vi "TestExec.Print Label.vi"(5 "CfgItem":string="URLLabel1", 6 "URL":string, 7 "CfgSection":string="Printer", 8 "error in":errorcluster, 10 "Text to Print":string, 11 "Config File":path) -> (0 "error out":errorcluster)   [LabVIEW 2018]
uses:
  <vilib>/Utility/config.llb/Read Key (String).vi
  <vilib>/httpClient/LabVIEWHTTPClient.lvlib
  <vilib>/Utility/config.llb/NI_LVConfig.lvlib
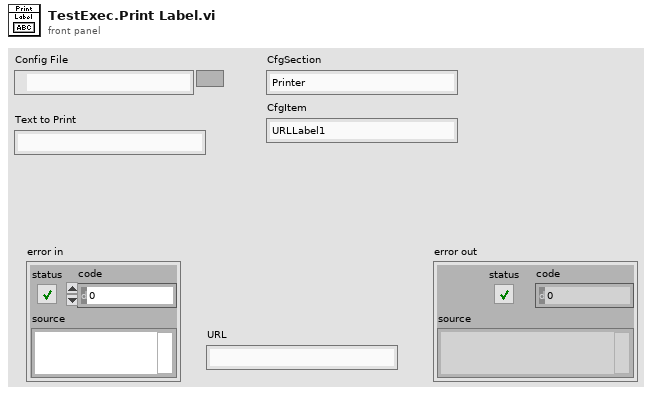
[diagram p1: front panel]
types:
  T1 = typedef "LabVIEWHTTPClient.lvlib/ClientHandle.ctl" = refnum<k1>
  T2 = typedef "NI_LVConfig.lvlib/Config Data RefNum.ctl" = refnum<k1>
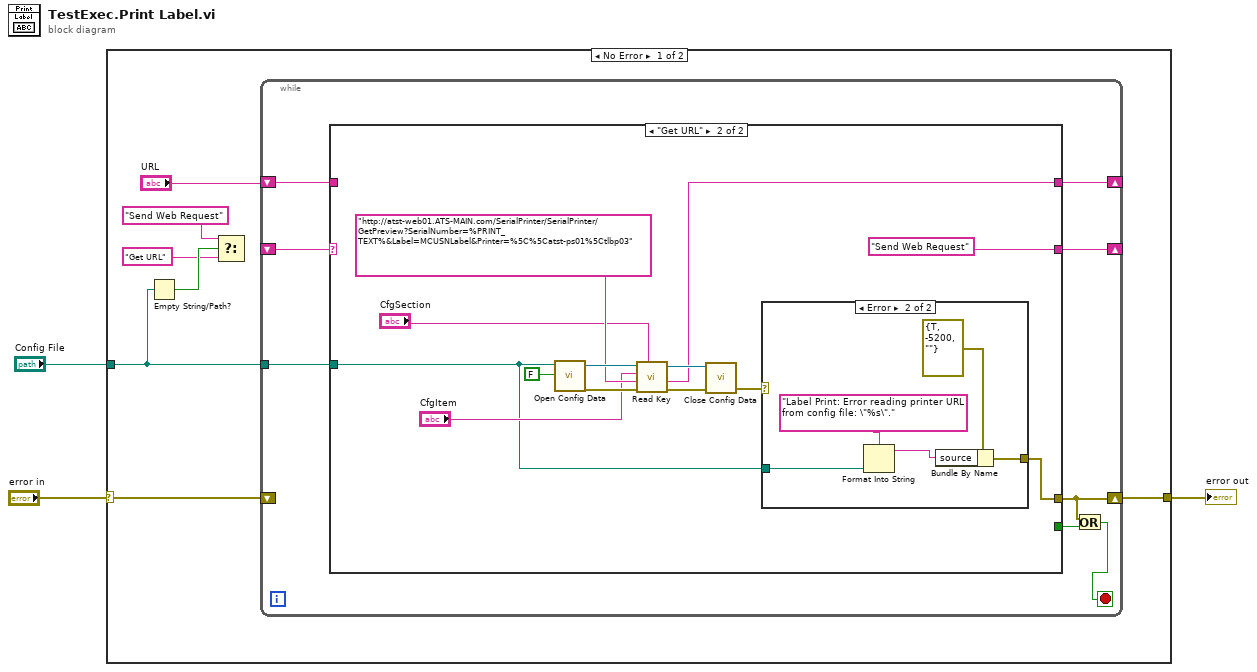
[diagram p0: block diagram]
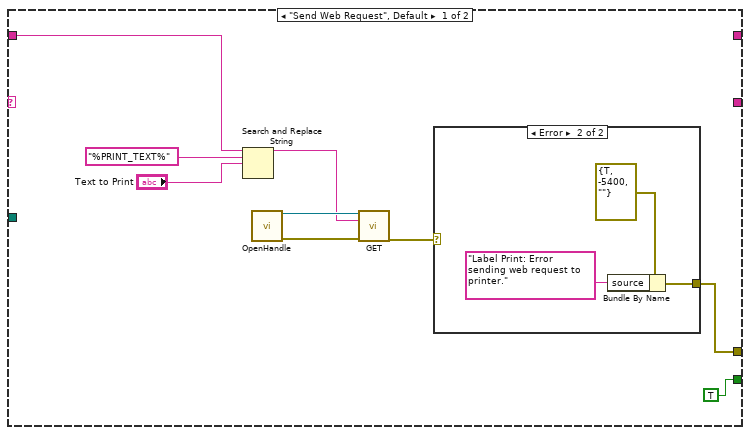
[diagram p2: hidden frame]
diagram:
  n1 = case shown="No Error" "error in" {
    selector: "error in" -> [w9 w49]
    tunnel: [w10 w49] -> w3
    tunnel: "Config File" -> [w6 _]
    frame No Error {
      n2 = Empty String/Path?(string/path=w6) -> (empty?=w7:bool)
      n3 = Select(t="Send Web Request", s=w7, f="Get URL") -> ()  [unwired: 1 out]
      n4 = while {
        shift-right: [w16] -> _
        shift-left: _ -> [w17]
        shift-right: [w15] -> _
        shift-left: "URL" -> [w18]
        shift-right: [w14] -> w10
        shift-left: w9 -> [_]
        tunnel: w6 -> [w11]
        stop <- w12 stop-if-true
        n5 = case shown="\"Get URL\"" w17 {
          tunnel: w18 -> [w26 _]
          tunnel: [_ "Send Web Request"] -> w16
          tunnel: [w20 w36] -> w14
          tunnel: [_ w35] -> w15
          tunnel: [TRUE _] -> w13
          tunnel: w11 -> [_ w31]
          frame "Send Web Request", Default {
            n6 = Search and Replace String(input string=w26, search string="%PRINT_TEXT%", replace string="Text to Print") -> (result string=w23:string)  [unwired: 5 in, 3 out]
            n7 = call <vilib>:"OpenHandle.vi"() -> ("client handle out"=w24:T1, "error out"=w25:errorcluster)  [unwired: 14 in]
            n8 = call <vilib>:"GET.vi"("client handle"=w24, "url"=w23, "error in (no error)"=w25) -> ("error out"=w21:errorcluster)  [unwired: 9 in, 3 out]
            n9 = case shown="Error" w21 {
              tunnel: [_ w29] -> w20
              frame No Error {
              }
              frame Error {
                n10 = Bundle By Name(cluster=errorcluster {"status"=TRUE, "code"=-5400, "source"=""} ("error constant"), "source"="Label Print: Error sending web request to printer.") -> (w29:errorcluster)
              }
            }
          }
          frame "Get URL" {
            n11 = call <vilib>:"Open Config Data.vi"("create file if necessary (T)"=FALSE, "configuration file path"=w31) -> ("error out"=w40:errorcluster, "refnum"=w41:T2)  [unwired: 7 in, 1 out]
            n12 = call-poly <vilib>:"Read Key.vi"("section"="CfgSection", "error in (no error)"=w40, "default value"="http://atst-web01.ATS-MAIN.com/SerialPrinter/SerialPrinter/GetPreview?SerialNumber=%PRINT_TEXT%&Label=MCUSNLabel&Printer=%5C%5Catst-ps01%5Ctlbp03", "key"="CfgItem", "refnum"=w41) -> ("error out"=w43:errorcluster, "value"=w35:string, "refnum out"=w42:T2)  [unwired: 3 in, 1 out]
            n13 = call <vilib>:"Close Config Data.vi"("error in (no error)"=w43, "refnum"=w42) -> ("error out"=w37:errorcluster)  [unwired: 8 in, 1 out]
            n14 = case shown="Error" w37 {
              tunnel: w31 -> [_ w45]
              tunnel: [_ w44] -> w36
              frame No Error {
              }
              frame Error {
                n15 = Format Into String(format string="Label Print: Error reading printer URL from config file: \"%s\".", w45) -> (resulting string=w46:string)  [unwired: 2 in, 1 out]
                n16 = Bundle By Name(cluster=errorcluster {"status"=TRUE, "code"=-5200, "source"=""} ("error constant"), "source"=w46) -> (w44:errorcluster)
              }
            }
          }
        }
        n17 = Or(x=w14, y=w13) -> (x .or. y?=w12:bool)
      }
    }
    frame Error {
    }
  }
  "error out" <- w3
